vi "Unpack 32I12's Packed into 24xI16 as 32xI16_Aligned.vi"(7 "Skip Error Check":bool, 8 "Error In":errorcluster, 11 "Input Array":i16[](array[numeric])) -> (0 "Error Out":errorcluster, 3 "Output Array":i16[](array[numeric]))   [LabVIEW 2012]
uses:
  <vilib>/Utility/tdmsutil.llb/TDMS Generate Random Data (I16).vi
  <userlib>/FlexRIO Host Library/FlexRIO Host API/Packer and Unpacker/32ch 12-bit Pack/Test Bench/ProcessingDLL/Release/ProcessingDLL.dll
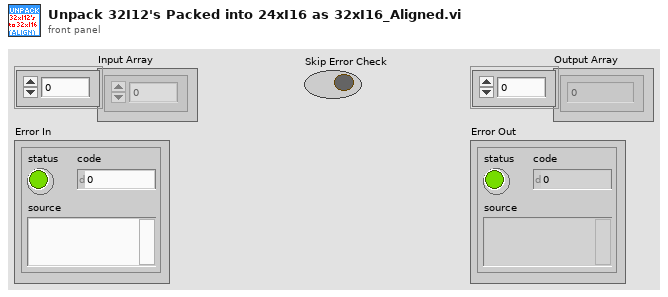
[diagram p1: front panel]
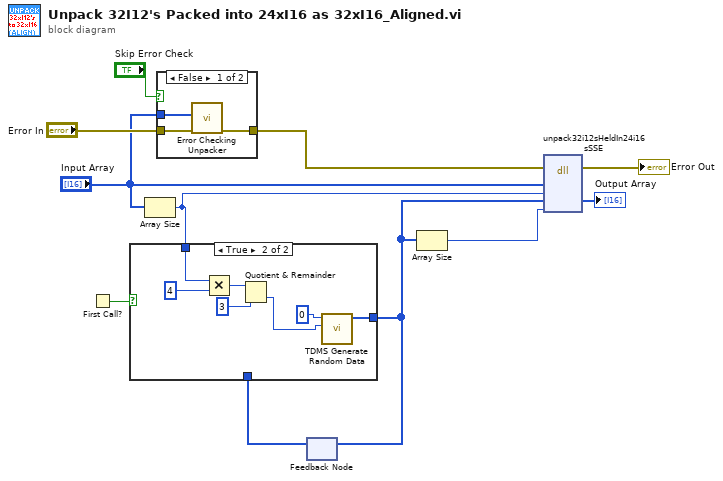
[diagram p0: block diagram]
diagram:
  n1 = First Call?() -> (First Call?: T/F=w11:bool)
  n2 = Array Size(array="Input Array") -> (size(s)=w10:i32)
  n3 = case shown="False" "Skip Error Check" {
    tunnel: "Error In" -> [w14 w15]
    tunnel: "Input Array" -> [w13 _]
    tunnel: [w12 w15] -> w2
    frame False {
      n4 = call <userlib>:"Error Checking Unpacker.vi"("error in"=w14, "packed i12s"=w13) -> ("error out"=w12:errorcluster)  [unwired: 9 in]
    }
    frame True {
    }
  }
  n5 = feedback #1() -> (w6:i16[])  [unwired: 1 in]
  n6 = case shown="True" w11 {
    tunnel: w10 -> [_ w22]
    tunnel: [w16 w17] -> w7
    tunnel: w6 -> [w16 _]
    frame False {
    }
    frame True {
      n7 = Multiply(x=w22, y=4) -> (x*y=w20:i32)
      n8 = Quotient & Remainder(x=w20, y=3) -> (floor(x/y)=w18:i32)  [unwired: 1 out]
      n9 = call-poly <vilib>:"TDMS Generate Random Data.vi"("number of samples"=w18, "data type"=i16 0) -> ("data"=w17:i16[])  [unwired: 8 in, 1 out]
    }
  }
  n10 = feedback-in #1(w7) -> ()
  n11 = Array Size(array=w7) -> (size(s)=w9:i32)
  n12 = dll-call lib="C:/Program Files (x86)/National Instruments/LabVIEW 2012/user.lib/FlexRIO Host Library/FlexRIO Host API/Packer and Unpacker/32ch 12-bit Pack/Test Bench/ProcessingDLL/Release/ProcessingDLL.dll" fn="unpack32i12sHeldIn24i16sSSE"(error in=w2, "source"="Input Array", "sourceSize"=w10, "destination"=w7, "destinationSize"=w9) -> (error out=→"Error Out":errorcluster, "destination"=→"Output Array":i16[])  [unwired: 6 in, 1 out]
